vi "main(Test DQMH modules).vi"() -> ()   [LabVIEW 2018, in "Application.lvlib"] (continued)
                n7427 = To Variant(anything=T4."demux1_10_channel10" ("demux1_10(x6)_encode")) -> (Variant=w15778:variant)
                n7428 = To Variant(anything=bool[] [FALSE, FALSE, FALSE, FALSE, FALSE, TRUE]) -> (Variant=w15793:variant)
                n7429 = Bundle By Name(cluster=w15784, "command"="MEAS.AllRelaysOFF") -> (w15792:T9)
                n7430 = Bundle By Name(cluster=w15784, "command"="MEAS.mux10-1", "data"=w15782) -> (w15775:T9)
                n7431 = Bundle By Name(cluster=w15784, "command"="MEAS.demux1-10", "data"=w15778) -> (w15776:T9)
                n7432 = Bundle By Name(cluster=w15784, "command"="MEAS.eMIC", "data"=w15793) -> (w15777:T9)
                n7433 = Build Array(w15792, w15775, w15776, w15777) -> (w15770:T9[])
                n7434 = To Variant(anything=w15774) -> (Variant=w15773:variant)
                n7435 = To Variant(anything=w15774) -> (Variant=w15772:variant)
                n7436 = Bundle By Name(cluster=w15771, "command"="MEAS.requestAC", "data"=w15773) -> (w15790:T9)
                n7437 = Bundle By Name(cluster=w15771, "command"="Apps.WaitForEvent", "data"=w15772) -> (w15786:T9)
                n7438 = Bundle By Name(cluster=w15771, "command"="Apps.UI Update 1") -> (w15787:T9)
                n7439 = Bundle By Name(cluster=w15771, "command"="WaitFor") -> (w15769:T9)
                n7440 = Build Array (concatenate)(w15770, w15769, w15790, w15786, w15787) -> (w15785:T9[])
              }
              frame True {
                w15800 = T9 {"command"="", "data"=variant} ("element")
                w15822 = T9 {"command"="", "data"=variant} ("element")
                n7441 = To Variant(anything=T3."mux10_1_channel10" ("mux10_1(x6)_encode")) -> (Variant=w15829:variant)
                n7442 = To Variant(anything=T2."mux6_1_channel6_3" ("mux6_1(3wires)_encode")) -> (Variant=w15827:variant)
                n7443 = To Variant(anything=T4."demux1_10_channel10" ("demux1_10(x6)_encode")) -> (Variant=w15823:variant)
                n7444 = To Variant(anything=bool[] [FALSE, FALSE, FALSE, FALSE, FALSE, TRUE]) -> (Variant=w15819:variant)
                n7445 = Bundle By Name(cluster=w15822, "command"="MEAS.AllRelaysOFF") -> (w15818:T9)
                n7446 = Bundle By Name(cluster=w15822, "command"="MEAS.mux10-1", "data"=w15829) -> (w15817:T9)
                n7447 = Bundle By Name(cluster=w15822, "command"="MEAS.mux6_1", "data"=w15827) -> (w15816:T9)
                n7448 = Bundle By Name(cluster=w15822, "command"="MEAS.demux1-10", "data"=w15823) -> (w15815:T9)
                n7449 = Bundle By Name(cluster=w15822, "command"="MEAS.eMIC", "data"=w15819) -> (w15814:T9)
                n7450 = Build Array(w15818, w15817, w15816, w15815, w15814) -> (w15799:T9[])
                n7451 = To Variant(anything=w15804) -> (Variant=w15802:variant)
                n7452 = To Variant(anything=w15804) -> (Variant=w15801:variant)
                n7453 = Bundle By Name(cluster=w15800, "command"="WaitFor") -> (w15798:T9)
                n7454 = Bundle By Name(cluster=w15800, "command"="MEAS.DMM dual read") -> (w15811:T9)
                n7455 = Bundle By Name(cluster=w15800, "command"="MEAS.requestAC", "data"=w15802) -> (w15810:T9)
                n7456 = Bundle By Name(cluster=w15800, "command"="Apps.WaitForEvent", "data"=w15801) -> (w15805:T9)
                n7457 = Bundle By Name(cluster=w15800, "command"="Apps.UI Update 1") -> (w15806:T9)
                n7458 = Build Array (concatenate)(w15799, w15798, w15811, w15810, w15805, w15806) -> (w15803:T9[])
              }
            }
          }
          frame True {
            n7459 = Bundle By Name(cluster=T9 {"command"="", "data"=variant} ("element"), "command"="Apps.UI Update 1") -> (w15833:T9)
            n7460 = Build Array(w15833) -> (w15832:T9[])
          }
        }
        n7461 = for {
          tunnel: w15748 -> [w15843] mode=indexing
          tunnel: w15756 -> [w15844]
          tunnel: [w15840] -> w15758 mode=indexing
          n7462 = Unbundle By Name(w15843) -> ("command"=w15842:string, "data"=w15841:variant)
          n7463 = call "App enquece.vi"("command data"=w15841, "command"=w15842, "queue in"=w15844) -> ("error out"=w15840:errorcluster)  [unwired: 7 in, 1 out]
        }
        n7464 = Merge Errors(w15759, w15758) -> (w15757:errorcluster)
      }
    }
    "DC Measure Completed" <- w237
    "Progress Status" <- w234
    n7465 = feedback-in #1(w234) -> ()
    n7466 = disable-structure shown="LOGGING==TRUE" {
      disable-tunnel: [w261 _] -> w235
      disable-tunnel: w236 -> [w259 _]
      frame condition #0 (active) {
        n7467 = call "string log (SubVI).vi"("error in (no error)"=w259, "Enum(log)"=enum16{"Init", "Log", "Read", "Clear"}."Read") -> ("error out"=w261:errorcluster, "State log"=→"State log":string)  [unwired: 8 in]
      }
      frame condition #1 {
      }
    }
  }
  n7468 = Release Queue(queue=w90, error in (no error)=w89) -> (error out=w8:errorcluster)  [unwired: 1 in, 2 out]
  n7469 = Unregister For Events(event registration refnum=w94) -> (error out=w10:errorcluster)  [unwired: 1 in]
  n7470 = Destroy User Event(user event=w7, error in=w8) -> (error out=w4:errorcluster)
  n7471 = while {
    shift-right: [w15849] -> w3
    shift-left: w5 -> [w15851]
    shift-right: [w15846] -> w2
    shift-left: w4 -> [w15850]
    stop <- w15847 stop-if-true
    n7472 = Get Queue Status(queue=w15851, error in (no error)=w15850) -> (queue out=w15849:refnum<queue>, error out=w15846:errorcluster, # elements in queue=w15848:i32)  [unwired: 1 in, 5 out]
    n7473 = Equal To 0?(x=w15848) -> (x = 0?=w15847:bool)
    n7474 = Wait (ms)(milliseconds to wait=u32 10) -> ()  [unwired: 1 out]
  }
  n7475 = Release Queue(queue=w3, error in (no error)=w2) -> (error out=w1:errorcluster)  [unwired: 1 in, 2 out]
  n7476 = Merge Errors(w10, w1) -> (w9:errorcluster)
  n7477 = disable-structure shown="RUN_TIME_ENGINE==True" {
    disable-tunnel: w9 -> [w15852 _]
    frame condition #0 (active) {
      "error out" <- w15852
    }
    frame condition #1 {
      n7478 = Quit LabVIEW(quit? (T)=TRUE) -> ()
    }
  }
